vi "Open Stream (FW7).vi"(6 "Axis Numbers (1, 2)":string[](array[string])=["1", "2"], 7 "Buffer Number (0)":u8, 8 "error in (no error)":errorcluster, 9 "Device Number":string, 10 "Stream Number (1)":u8=1, 11 "VISA resource name":refnum<visa-resource-name>) -> (0 "error out":errorcluster, 3 "VISA resource name out":refnum<visa-resource-name>)   [LabVIEW 2015, in "Zaber A Series.lvlib"]
doc: "Opens a stream for receiving coordinated motion commands. \n\nUse zero as the buffer number to open a live stream that will execute commands immediately, or to record commands for later execution specify a buffer number between 1 and the value of the \"stream.numbufs\" setting, which is returned by the Get Stream Support Info VI.\n\nFor a live stream you must specify one or more axis numbers to execute the commands on. If your device has Firmware version 7, you can add the word \"lockstep\" before the number to specify an existing lockstep group instead of a single axis. For example \"lockstep 1\" will use lockstep group 1 instead of axis 1.\n\nFor a buffered stream the axis numbers are ignored until you invoke the buffer, but the quantity of them still matters at stream open time.\n\nTo invoke a buffered stream you must open a live stream (and specify the actual axis numbers) and then invoke the buffer using the Call Stream VI.\n\nThis VI does not check in advance for error conditions such as streams not being supported.\n\nThis VI requires that the Initialize VI has been called with the same serial port."
uses:
  Zaber A Series.lvlib
  Private/All Commands.ctl
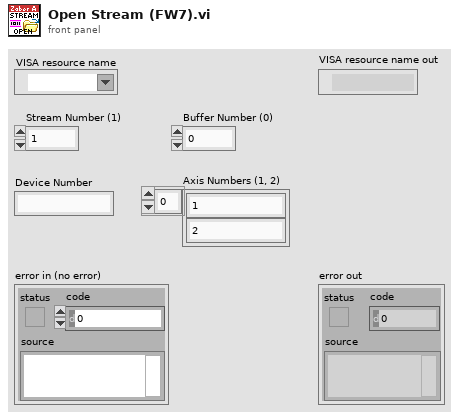
[diagram p1: front panel]
types:
  T1 = typedef "Zaber A Series.lvlib/All Commands.ctl" = string
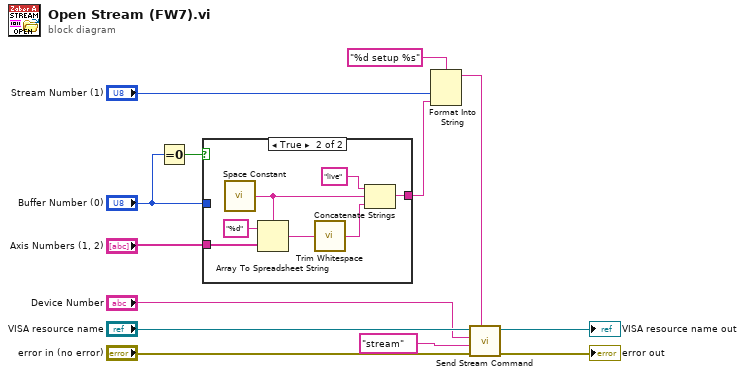
[diagram p0: block diagram]
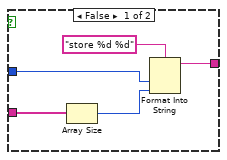
[diagram p2: hidden frame]
diagram:
  n1 = Equal To 0?(x="Buffer Number (0)") -> (x = 0?=w11:bool)
  n2 = case shown="True" w11 {
    tunnel: "Axis Numbers (1, 2)" -> [w18 w22]
    tunnel: [w14 w21] -> w7
    tunnel: "Buffer Number (0)" -> [w15 _]
    frame False {
      n3 = Array Size(array=w18) -> (size(s)=w16:i32)
      n4 = Format Into String(format string="store %d %d", w15, w16) -> (resulting string=w14:string)  [unwired: 2 in, 1 out]
    }
    frame True {
      n5 = call <vilib>:"Space Constant.vi"() -> ("String"=w25:string)
      n6 = Array To Spreadsheet String(delimiter (Tab)=w25, array=w22, 3:"%d" ("format string")) -> (spreadsheet string=w20:string)
      n7 = call <vilib>:"Trim Whitespace.vi"("string"=w20) -> ("trimmed string"=w19:string)  [unwired: 1 in]
      n8 = Concatenate Strings("live", w25, w19) -> (w21:string)
    }
  }
  n9 = Format Into String(format string="%d setup %s", "Stream Number (1)", w7) -> (resulting string=w6:string)  [unwired: 2 in, 1 out]
  n10 = call "Send Stream Command.vi"("Data"=w6, "error in (no error)"="error in (no error)", "Command"=T1 "stream" ("Complete Command List"), "Device Number"="Device Number", "VISA resource name"="VISA resource name") -> ("error out"=→"error out":errorcluster, "VISA resource name out"=→"VISA resource name out":refnum<visa-resource-name>)  [unwired: 5 in]
